vi "Error Codes List Window.vi"(5 "shift pressed?":bool, 7 "project file":path, 8 "error in (no error)":errorcluster, 9 "combo box text":string, 10 "scripting templates directory":path, 11 "project error file":path) -> ()   [LabVIEW 2017]
uses:
  Controls/Error Codes List Window Data.ctl
  Controls/Error Codes List Window States.ctl
  Controls/Quick Drop Input.ctl
  Controls/Error Codes List Window References.ctl
  Controls/Flags.ctl
  Error List/Scope.ctl
  Error List/Error Owner and ID.ctl
  <vilib>/Utility/miscctls.llb/LVRowAndColumnUnsignedTypeDef.ctl
  Controls/Themes.ctl
  Controls/Error Code Window Modes.ctl
  <vilib>/Utility/SystemLogging/NI_SystemLogging.lvlib
  Error File Management/Error File Management.lvlib
panel:
  in  "error codes":i32(listbox)
  out "loading":u8(ring)
  in  "edit error":bool
  in  "add error":bool
  in  "remove error":bool
  in  "edit file":bool
  in  "scope":bool
  in  "cancel":bool
  in  "ok":bool
  in  "filter":bool
  in  "filter string":string
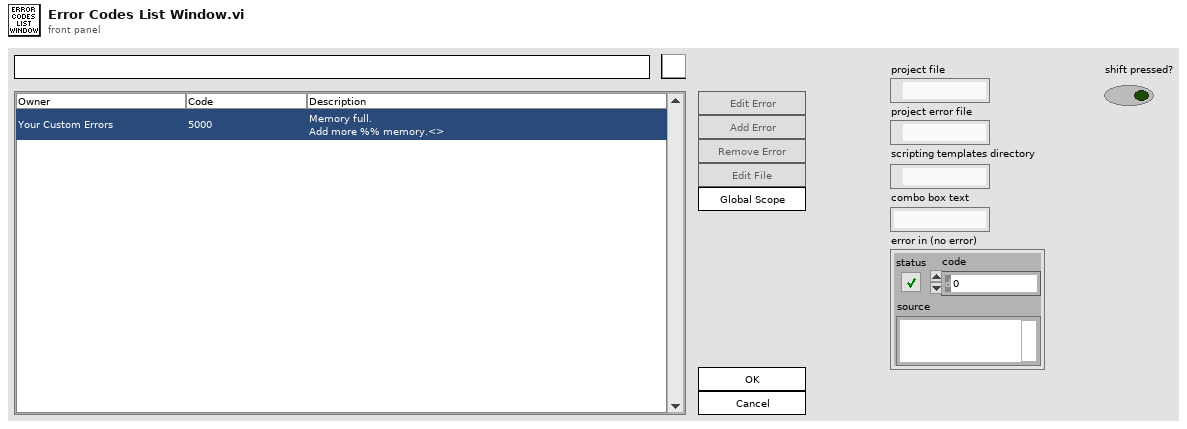
[diagram p1: front panel]
types:
  T1 = typedef "Error Codes List Window References.ctl" = cluster{"UI VI":refnum<vi>, "edit error":refnum<vi>, "add error":refnum<vi>, "remove error":refnum<vi>, "edit file":refnum<vi>, "scope":refnum<vi>, "ok":refnum<vi>, "cancel":refnum<vi>, "filter string":refnum<vi>, "filter":refnum<vi>, "error codes":refnum<vi>, "loading":refnum<vi>}
  T2 = typedef "Error Codes List Window Data.ctl" = cluster{"Q":refnum<queue>, "quick drop input":T3, "control references":T1, "flags":T4, "scope":T5, "error list":variant, "selected error":T6, "displayed errors":T6[]}
  T3 = typedef "Quick Drop Input.ctl" = cluster{"project file":path, "project error file":path, "scrip templates dir":path, "combo box string":string}
  T4 = typedef "Flags.ctl" = cluster{"place on cursor?":bool, "global scope loaded?":bool, "global modified?":bool, "filter on?":bool, "project scope avaiable?":bool, "shift pressed?":bool, "selected?":bool, "editable?":bool}
  T5 = typedef "Scope.ctl" = enum16{"project", "global"}
  T6 = typedef "Error Owner and ID.ctl" = cluster{"owner path":string, "ID":string}
  T7 = typedef "Error Codes List Window States.ctl" = enum16{"init", "load project errors", "parse combo box", "update list view", "open FP", "close", "idle", "add error", "remove error", "edit error", "edit file", "change scope", "filter"}
  T8 = enum32{"Invalid", "Standard", "Closed", "Hidden", "Minimized", "Maximized"}
  T9 = typedef "Themes.ctl" = enum16{"init", "edit buttons disable state", "loading on", "loading off", "scope name"}
  T10 = typedef "LVRowAndColumnUnsignedTypeDef.ctl" = cluster{"Row":u32, "Column":u32}
  T11 = typedef "Error File Management.lvlib/NI Error.ctl" = errorcluster
  T12 = typedef "LVPoint32TypeDef.ctl" = cluster{"Horizontal":i32, "Vertical":i32}
  T13 = typedef "Error Code Window Modes.ctl" = u8
  T14 = typedef "Error Code File Properties.ctl" = cluster{"path":path, "simplified path":string, "name":string, "display name":string, "family name":string, "comment":string, "parsable?":bool, "file modified?":bool}
  T15 = cluster{"new element/subarray":T14, "errors":T11[]}[]
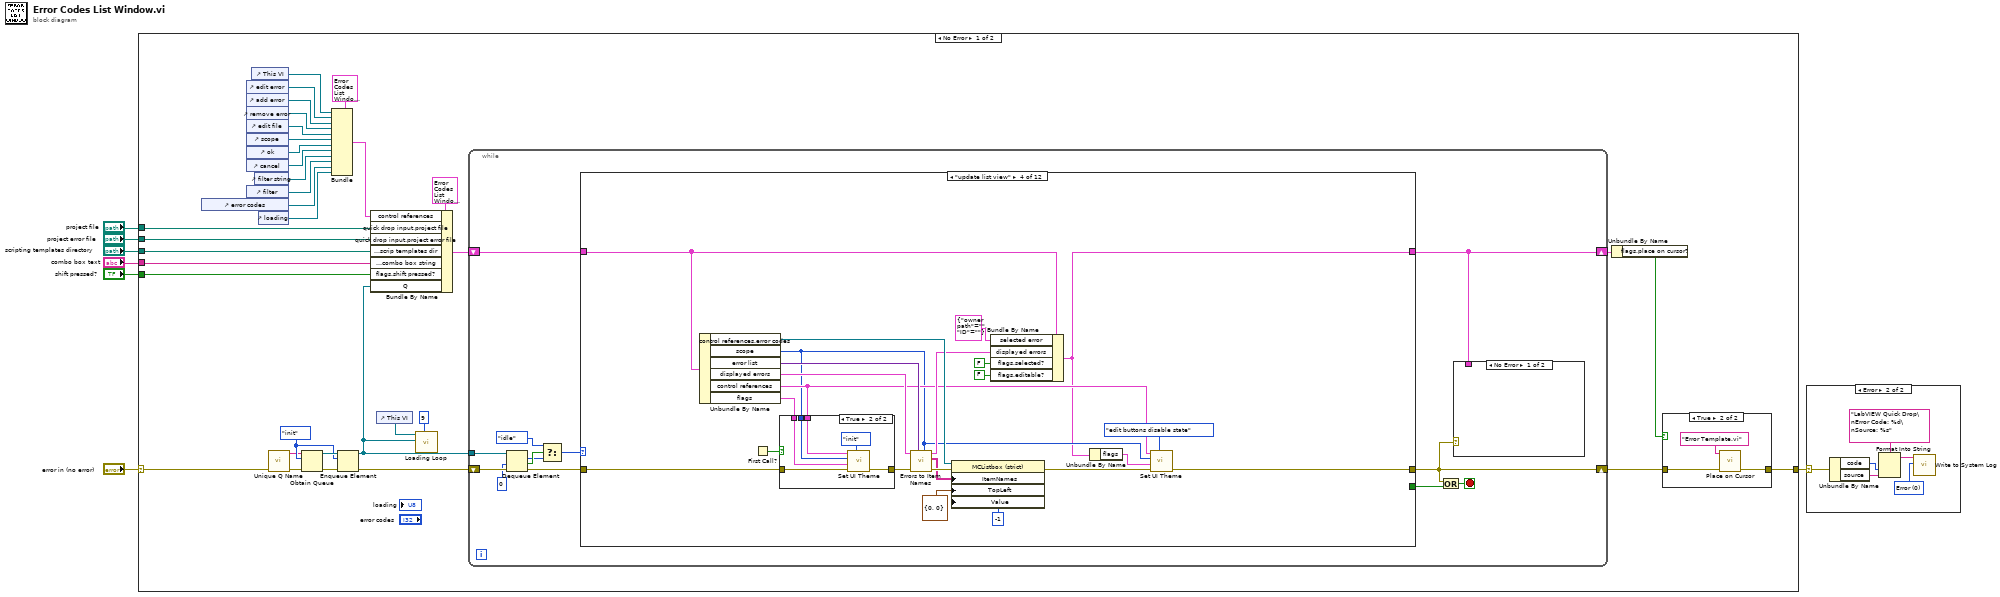
[diagram p0: block diagram]
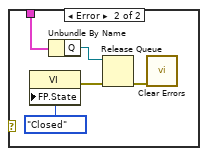
[diagram p2: hidden frame]
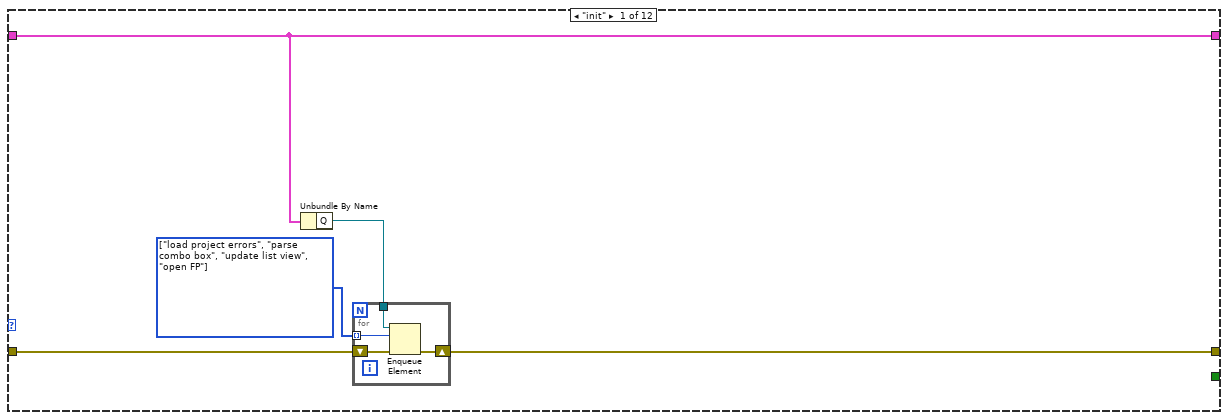
[diagram p3: hidden frame]
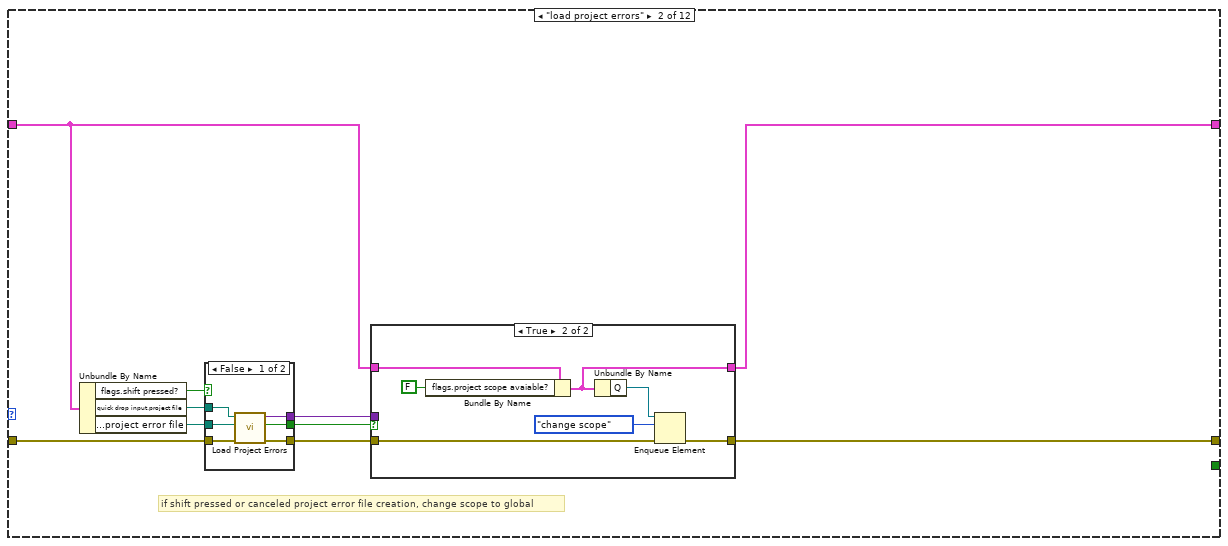
[diagram p4: hidden frame]
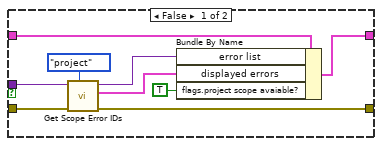
[diagram p6: hidden frame]
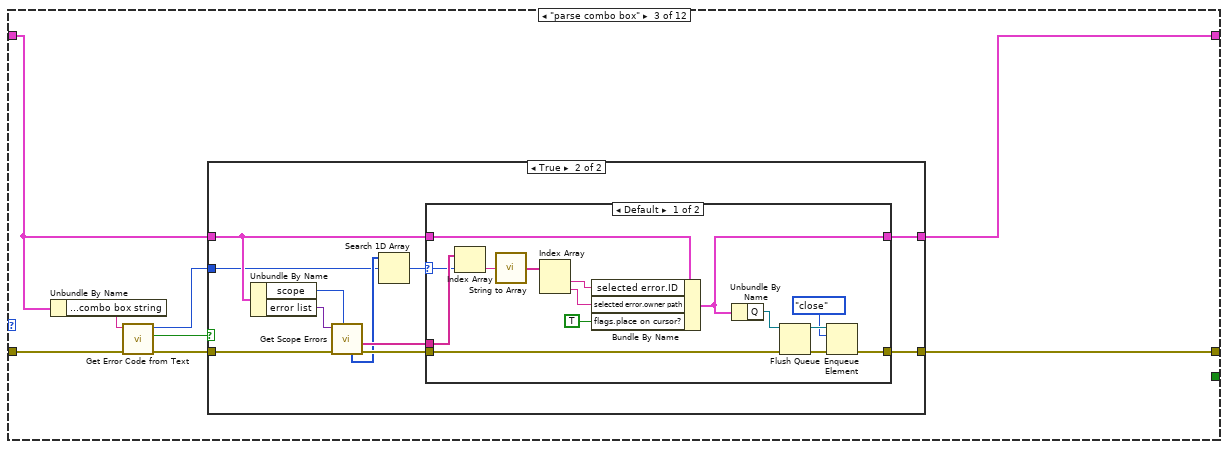
[diagram p7: hidden frame]
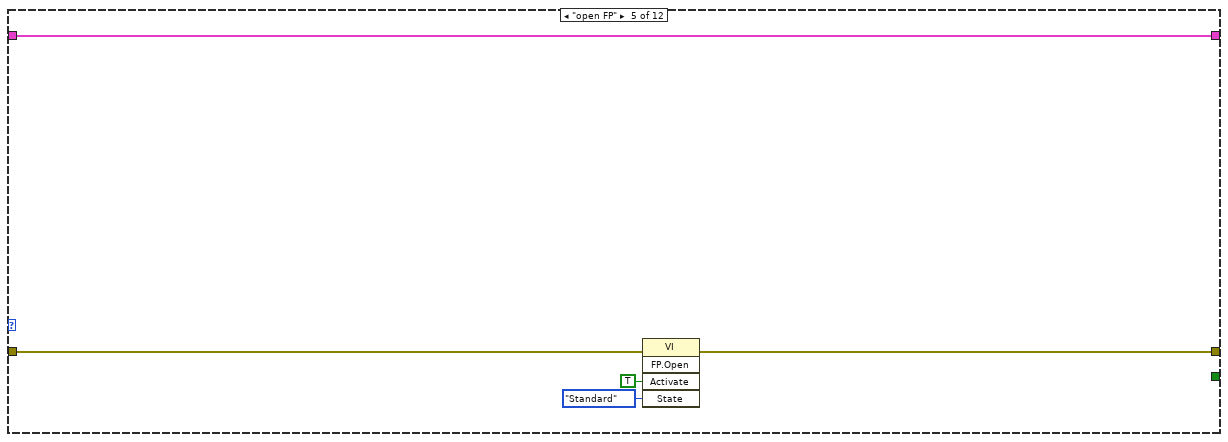
[diagram p11: hidden frame]
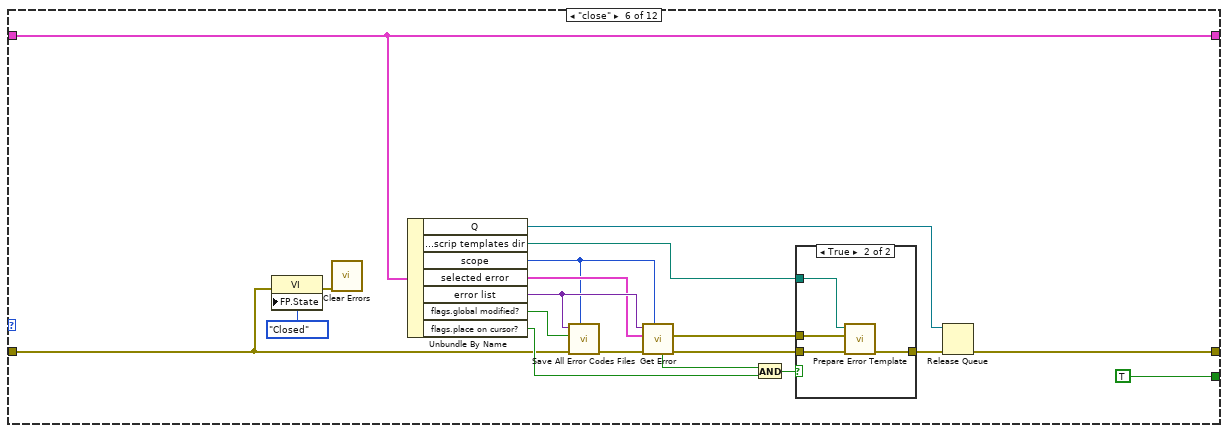
[diagram p12: hidden frame]
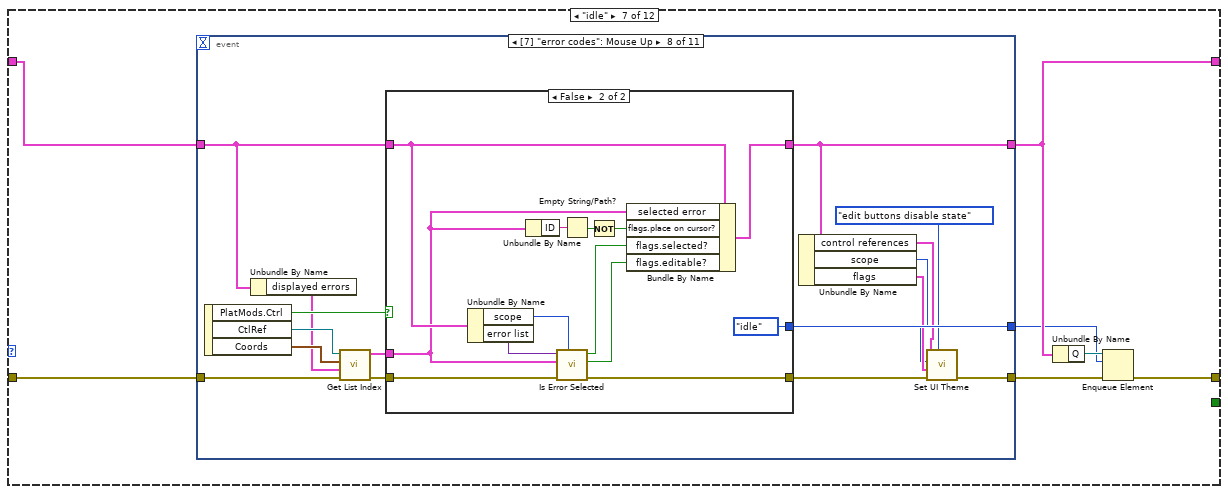
[diagram p14: hidden frame]
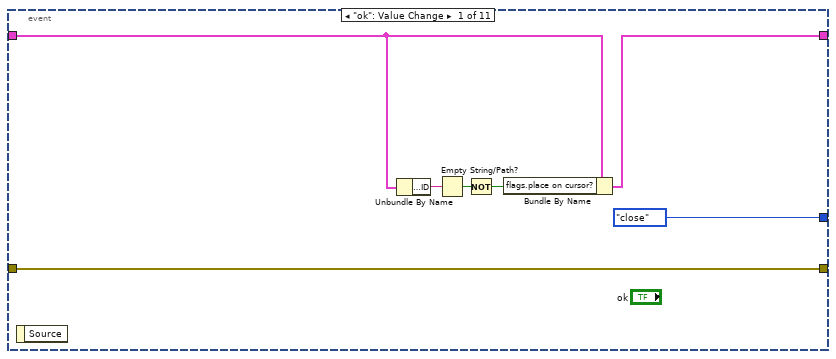
[diagram p15: hidden frame]
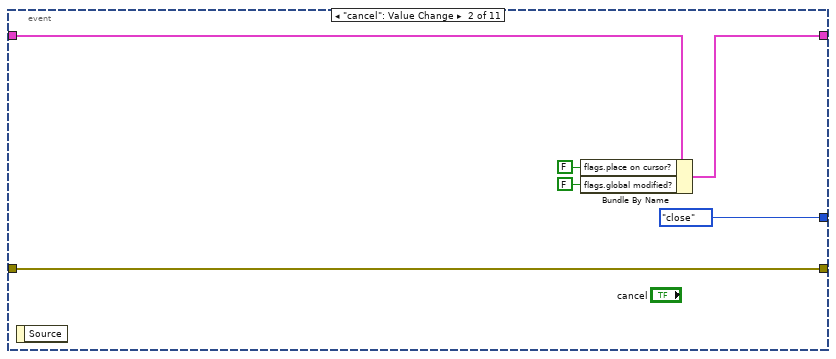
[diagram p16: hidden frame]
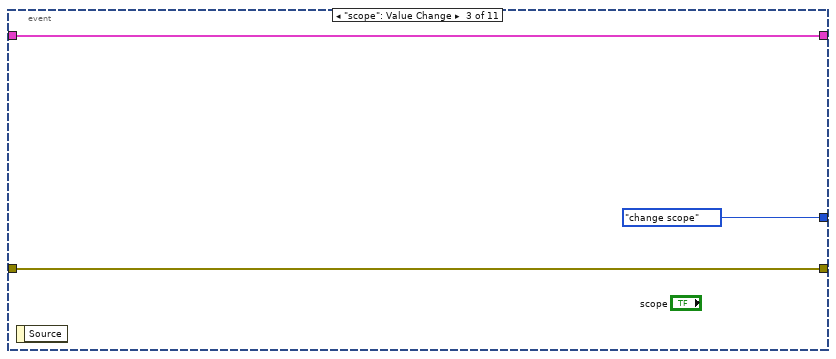
[diagram p17: hidden frame]
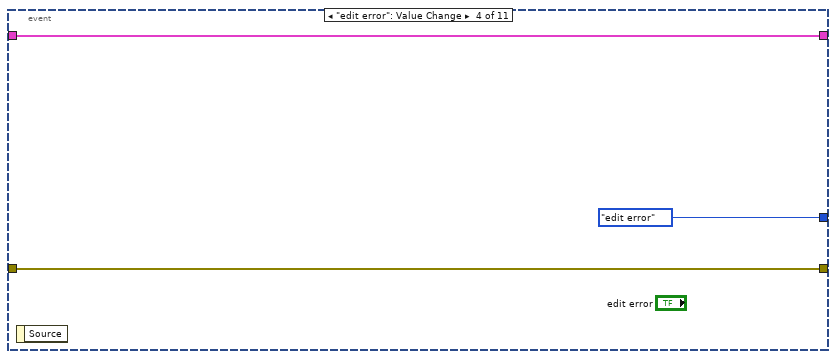
[diagram p18: hidden frame]
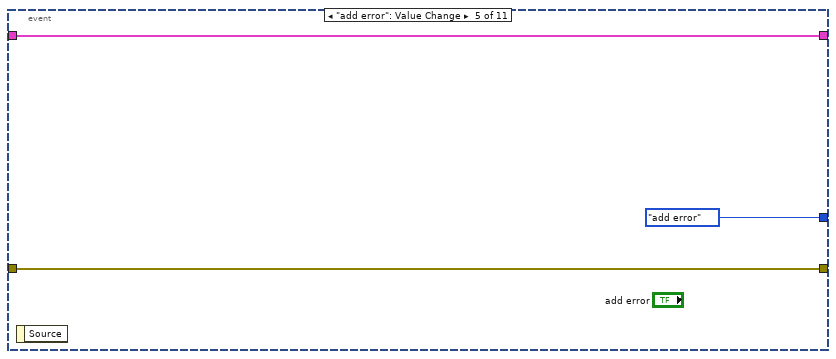
[diagram p19: hidden frame]
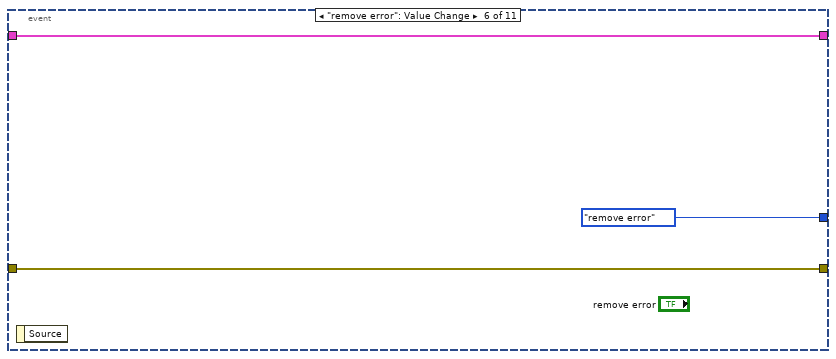
[diagram p20: hidden frame]
diagram:
  n1 = case shown="No Error" "error in (no error)" {
    selector: "error in (no error)" -> [w29 w440]
    tunnel: "project error file" -> [w12 _]
    tunnel: "scripting templates directory" -> [w27 _]
    tunnel: [w39 w440] -> w6
    tunnel: "combo box text" -> [w26 _]
    tunnel: "project file" -> [w11 _]
    tunnel: "shift pressed?" -> [w8 _]
    frame No Error {
      w30 = Error_Codes_List_Window_States."init" ("states")
      n2 = control-ref of="error codes"() -> (w15:refnum<vi>)
      n3 = control-ref of="edit error"() -> (w24:refnum<vi>)
      n4 = control-ref of="add error"() -> (w23:refnum<vi>)
      n5 = control-ref of="remove error"() -> (w22:refnum<vi>)
      n6 = control-ref of="edit file"() -> (w21:refnum<vi>)
      n7 = control-ref of="scope"() -> (w20:refnum<vi>)
      n8 = control-ref of="ok"() -> (w19:refnum<vi>)
      n9 = control-ref of="cancel"() -> (w18:refnum<vi>)
      n10 = control-ref of="filter"() -> (w16:refnum<vi>)
      n11 = control-ref of="This VI"() -> (w10:refnum<vi>)
      n12 = control-ref of="filter string"() -> (w17:refnum<vi>)
      n13 = control-ref of="loading"() -> (w14:refnum<vi>)
      n14 = call "Unique Q Name.vi"() -> ("unique Q name"=w28:string)  [unwired: 11 in]
      n15 = Obtain Queue(name (unnamed)=w28, element data type=w30, error in (no error)=w29) -> (queue out=w33:refnum<queue>, error out=w32:errorcluster)  [unwired: 2 in, 1 out]
      n16 = Bundle(cluster=T1 {"UI VI"=refnum, "edit error"=refnum, "add error"=refnum, "remove error"=refnum, "edit file"=refnum, "scope"=refnum, "ok"=refnum, "cancel"=refnum, "filter string"=refnum, "filter"=refnum, "error codes"=refnum, "loading"=refnum} ("control references"), "UI VI"=w10, "edit error"=w24, "add error"=w23, "remove error"=w22, "edit file"=w21, "scope"=w20, "ok"=w19, "cancel"=w18, "filter string"=w17, "filter"=w16, "error codes"=w15, "loading"=w14) -> (w13:T1)
      n17 = Enqueue Element(queue=w33, element=w30, error in (no error)=w32) -> (queue out=w25:refnum<queue>, error out=w31:errorcluster)  [unwired: 1 in, 1 out]
      n18 = Bundle By Name(cluster=T2 {"Q"=refnum, "quick drop input"={"project file"=path "", "project error file"=path "", "scrip templates dir"=path "", "combo box string"=""}, "control references"={"UI VI"=refnum, "edit error"=refnum, "add error"=refnum, "remove error"=refnum, "edit file"=refnum, "scope"=refnum, "ok"=refnum, "cancel"=refnum, "filter string"=refnum, "filter"=refnum, "error codes"=refnum, "loading"=refnum}, "flags"={"place on cursor?"=FALSE, "global scope loaded?"=FALSE, "global modified?"=FALSE, "filter on?"=FALSE, "project scope avaiable?"=FALSE, "shift pressed?"=FALSE, "selected?"=FALSE, "editable?"=FALSE}, "scope"=enum."project", "error list"=variant(cluster{"properties":cluster{"path":path, "simplified path":string, "name":string, "parsable?":bool, "project?":bool}, "data":cluster{"family":cluster{"family name":string, "display name":string}, "comment":string, "project errors":cluster{"error cluster":errorcluster, "owner file path":path, "owner display name":string, "parsable?":bool}[]}, "file modified?":bool}[] []), "selected error"={"owner path"="", "ID"=""}, "displayed errors"=[]} ("output cluster"), "control references"=w13, "quick drop input.project file"=w11, "quick drop input.project error file"=w12, "quick drop input.scrip templates dir"=w27, "quick drop input.combo box string"=w26, "flags.shift pressed?"=w8, "Q"=w25) -> (w40:T2)
      n19 = control-ref of="This VI"() -> (w35:refnum<vi>)
      n20 = call "Loading Loop.vi"("ctrl index"=9, "Q"=w25, "owner VI"=w35) -> ()  [unwired: 9 in]
      n21 = while {
        shift-right: [w43] -> w38
        shift-left: w31 -> [w51]
        shift-right: [w42] -> w37
        shift-left: w40 -> [w52]
        tunnel: w25 -> [w49]
        stop <- w53 stop-if-true
        n22 = Dequeue Element(queue=w49, timeout in ms (-1)=0, error in (no error)=w51) -> (element=w46:T7, timed out?=w47:bool, error out=w50:errorcluster)  [unwired: 1 out]
        n23 = Select(t=Error_Codes_List_Window_States."idle", s=w47, f=w46) -> (s? t:f=w45:T7)
        n24 = case shown="\"update list view\"" w45 {
          selector: w45 -> [_ _ _ _ _ _ _ _ w317 _ _ _]
          tunnel: [_ _ _ _ _ TRUE _ _ _ _ _ _] -> w54
          tunnel: w50 -> [w64 w78 w110 w158 w172 w179 w206 w311 w328 w351 w385 w421]
          tunnel: [w60 w70 w103 w148 w175 w192 w202 w301 w320 w339 w364 w411] -> w43
          tunnel: w52 -> [w63 w74 w106 w155 w171 w189 w205 w309 w327 w350 w384 w420]
          tunnel: [w63 w77 w105 w142 w171 w189 w201 w310 w326 w344 w378 w422] -> w42
          frame "init" {
            w61 = T7[] [enum."load project errors", enum."parse combo box", enum."update list view", enum."open FP"] items=["init", "load project errors", "parse combo box", "update list view", "open FP", "close", "idle", "add error", "remove error", "edit error", "edit file", "change scope", "filter"] ("t")
            n25 = Unbundle By Name(w63) -> ("Q"=w62:refnum<queue>)
            n26 = for {
              tunnel: w62 -> [w67]
              shift-right: [w68] -> w60
              shift-left: w64 -> [w66]
              tunnel: w61 -> [w65] mode=indexing
              n27 = Enqueue Element(queue=w67, element=w65, error in (no error)=w66) -> (error out=w68:errorcluster)  [unwired: 1 in, 2 out]
            }
          }
          frame "load project errors" {
            # "if shift pressed or canceled project error file creation, change scope to global"
            n28 = Unbundle By Name(w74) -> ("flags.shift pressed?"=w69:bool, "quick drop input.project file"=w72:path, "quick drop input.project error file"=w73:path)
            n29 = case shown="False" w69 {
              selector: w69 -> [_ w86]
              tunnel: w78 -> [w84 w85]
              tunnel: [w83 _] -> w76
              tunnel: [w82 w86] -> w75
              tunnel: w73 -> [w81 _]
              tunnel: w72 -> [w80 _]
              tunnel: [w79 w85] -> w71
              frame False {
                n30 = call "Load Project Errors.vi"("error in (no error)"=w84, "error file path"=w81, "project path"=w80) -> ("error out"=w79:errorcluster, "canceled?"=w82:bool, "error list <top>"=w83:variant)  [unwired: 6 in]
              }
              frame True {
              }
            }
            n31 = case shown="True" w75 {
              tunnel: [w95 w97] -> w77
              tunnel: w74 -> [w94 w98]
              tunnel: w76 -> [w93 _]
              tunnel: w71 -> [w91 w101]
              tunnel: [w90 w100] -> w70
              frame False {
                n32 = call "Get Scope Error IDs.vi"("scope"=Scope."project", "error in (no error)"=w91, "error list <top>"=w93) -> ("error out"=w90:errorcluster, "error IDs"=w89:T6[], "error list <top> dup"=w92:variant)  [unwired: 6 in]
                n33 = Bundle By Name(cluster=w94, "error list"=w92, "displayed errors"=w89, "flags.project scope avaiable?"=TRUE) -> (w95:T2)
              }
              frame True {
                n34 = Bundle By Name(cluster=w98, "flags.project scope avaiable?"=FALSE) -> (w97:T2)
                n35 = Unbundle By Name(w97) -> ("Q"=w102:refnum<queue>)
                n36 = Enqueue Element(queue=w102, element=Error_Codes_List_Window_States."change scope", error in (no error)=w101) -> (error out=w100:errorcluster)  [unwired: 1 in, 2 out]
              }
            }
          }
          frame "parse combo box" {
            n37 = Unbundle By Name(w106) -> ("quick drop input.combo box string"=w109:string)
            n38 = call "Get Error Code from Text.vi"("error in (no error)"=w110, "text"=w109) -> ("error out"=w104:errorcluster, "found?"=w108:bool, "code"=w107:i32)  [unwired: 7 in]
            n39 = case shown="True" w108 {
              tunnel: w107 -> [_ w113]
              tunnel: [w112 w122] -> w105
              tunnel: w106 -> [w112 w121]
              tunnel: w104 -> [w111 w118]
              tunnel: [w111 w119] -> w103
              frame False {
              }
              frame True {
                n40 = Unbundle By Name(w121) -> ("scope"=w115:T5, "error list"=w116:variant)
                n41 = call "Get Scope Errors.vi"("scope"=w115, "error in (no error)"=w118, "error list <top> in"=w116) -> ("error out"=w117:errorcluster, "attributes"=w123:string[], "error codes"=w114:i32[])  [unwired: 4 in, 2 out]
                n42 = Search 1D Array(1D array=w114, element=w113) -> (index of element=w120:i32)  [unwired: 1 in]
                n43 = case shown="Default" w120 {
                  selector: w120 -> [w128 _]
                  tunnel: [w133 w140] -> w122
                  tunnel: w121 -> [w137 w140]
                  tunnel: w117 -> [w132 w139]
                  tunnel: [w130 w139] -> w119
                  tunnel: w123 -> [w129 _]
                  frame Default {
                    n44 = Index Array(array=w129, index=w128) -> (element=w124:string)
                    n45 = call "String to Array.vi"("string"=w124) -> ("array"=w127:string[])  [unwired: 1 in]
                    n46 = Index Array(array=w127) -> (element #1=w126:string, element #2=w125:string)  [unwired: 2 in]
                    n47 = Bundle By Name(cluster=w137, "selected error.ID"=w126, "selected error.owner path"=w125, "flags.place on cursor?"=TRUE ("place on cursor?")) -> (w133:T2)
                    n48 = Unbundle By Name(w133) -> ("Q"=w136:refnum<queue>)
                    n49 = Flush Queue(queue=w136, error in (no error)=w132) -> (queue out=w135:refnum<queue>, error out=w131:errorcluster)  [unwired: 1 out]
                    n50 = Enqueue Element(queue=w135, element=Error_Codes_List_Window_States."close", error in (no error)=w131) -> (error out=w130:errorcluster)  [unwired: 1 in, 2 out]
                  }
                  frame -1 {
                  }
                }
              }
            }
          }
          frame "update list view" {
            n51 = Unbundle By Name(w155) -> ("control references.error codes"=w161:refnum<vi>, "scope"=w146:T5, "error list"=w159:variant, "displayed errors"=w160:T6[], "control references"=w147:T1, "flags"=w145:T4)
            n52 = First Call?() -> (First Call?: T/F=w151:bool)
            n53 = case shown="True" w151 {
              tunnel: w158 -> [w164 w170]
              tunnel: [w164 w169] -> w152
              tunnel: w146 -> [_ w168]
              tunnel: w147 -> [_ w167]
              tunnel: w145 -> [_ w166]
              frame False {
              }
              frame True {
                n54 = call "Set UI Theme.vi"("theme"=Themes."init", "error in (no error)"=w170, "flags"=w166, "global scope?"=w168, "control references"=w167) -> ("error out"=w169:errorcluster)  [unwired: 6 in]
              }
            }
            n55 = call "Errors to Item Names.vi"("scope"=w146, "error list <top>"=w159, "error in (no error)"=w152, "displayed errors in"=w160) -> ("error out"=w163:errorcluster, "item names"=w157:string[][], "displayed errors out"=w156:T6[])  [unwired: 5 in]
            n56 = property on="Property Node" class="MCListbox (strict)"(reference=w161, error in=w163, "ItemNames"=w157, "TopLeft"=T10 {"Row"=0, "Column"=0} ("Top Left Visible Cell"), "Value"=-1 ("error codes list")) -> (error out=w149:errorcluster)  [unwired: 1 out]
            n57 = Bundle By Name(cluster=w155, "selected error"=T6 {"owner path"="", "ID"=""}, "displayed errors"=w156, "flags.selected?"=FALSE, "flags.editable?"=FALSE) -> (w142:T2)
            n58 = Unbundle By Name(w142) -> ("flags"=w141:T4)
            n59 = call "Set UI Theme.vi"("theme"=Themes."edit buttons disable state", "error in (no error)"=w149, "flags"=w141, "global scope?"=w146, "control references"=w147) -> ("error out"=w148:errorcluster)  [unwired: 6 in]
          }
          frame "open FP" {
            n60 = invoke class="VI" method="FP.Open"(error in=w172, "Activate"=TRUE ("Activate?"), "State"=T8."Standard") -> (error out=w175:errorcluster)  [unwired: 2 in, 4 out]
          }
          frame "close" {
            n61 = property class="VI"(error in=w179, "FP.State"=T8."Closed" ("Front Panel Window:State")) -> (error out=w178:errorcluster)  [unwired: 1 in, 1 out]
            n62 = call <vilib>:"Clear Errors.vi"("error in (no error)"=w178) -> ()  [unwired: 5 in, 2 out]
            n63 = Unbundle By Name(w189) -> ("Q"=w191:refnum<queue>, "quick drop input.scrip templates dir"=w190:path, "scope"=w180:T5, "selected error"=w181:T6, "error list"=w184:variant, "flags.global modified?"=w187:bool, "flags.place on cursor?"=w183:bool)
            n64 = call "Save All Error Codes Files.vi"("scope"=w180, "error in (no error)"=w179, "save? (T)"=w187, "error list <top>"=w184) -> ("error out"=w186:errorcluster)  [unwired: 7 in]
            n65 = call "Get Error.vi"("scope"=w180, "error in (no error)"=w186, "owner error"=w181, "error list <top>"=w184) -> ("error out"=w185:errorcluster, "error"=w176:T11, "found?"=w177:bool)  [unwired: 3 in, 2 out]
            n66 = And(x=w177, y=w183) -> (x .and. y?=w182:bool)
            n67 = case shown="True" w182 {
              tunnel: w185 -> [w195 w199]
              tunnel: [w195 w198] -> w193
              tunnel: w190 -> [_ w197]
              tunnel: w176 -> [_ w196]
              frame False {
              }
              frame True {
                n68 = call "Prepare Error Template.vi"("error in (no error)"=w199, "error"=w196, "templates directory"=w197) -> ("error out"=w198:errorcluster)  [unwired: 8 in]
              }
            }
            n69 = Release Queue(queue=w191, error in (no error)=w193) -> (error out=w192:errorcluster)  [unwired: 1 in, 2 out]
          }
          frame "idle" {
            n70 = event shown="[7] \"error codes\": Mouse Up" {
              selector: _ -> [_ _ _ _ _ _ _ _ _ _ _]
              dyn-events: _ -> [_ _ _ _ _ _ _ _ _ _ _]
              timeout: _ -> [_ _ _ _ _ _ _ _ _ _ _]
              tunnel: w206 -> [w213 w217 w222 w225 w228 w231 w233 w249 w284 w290 w291]
              tunnel: [w213 w217 w222 w225 w228 w231 w233 w240 w284 w290 w291] -> w203
              tunnel: w205 -> [w210 w219 w221 w224 w227 w230 w234 w245 w280 w289 w295]
              tunnel: [w212 w218 w221 w224 w227 w230 w234 w238 w282 w289 w294] -> w201
              tunnel: [Error_Codes_List_Window_States."close" ("states") Error_Codes_List_Window_States."close" ("states") Error_Codes_List_Window_States."change scope" ("states") Error_Codes_List_Window_States."edit error" ("states") Error_Codes_List_Window_States."add error" ("states") Error_Codes_List_Window_States."remove error" ("states") Error_Codes_List_Window_States."edit file" ("states") w243 Error_Codes_List_Window_States."close" ("states") w285 Error_Codes_List_Window_States."filter" ("states")] -> w200
              event "ok": Value Change {
                n71 = event-data() -> ()  [unwired: 1 in, 1 out]
                n72 = Unbundle By Name(w210) -> ("selected error.ID"=w209:string)
                n73 = Empty String/Path?(string/path=w209) -> (empty?=w208:bool)
                n74 = Not(x=w208) -> (.not. x?=w207:bool)
                n75 = Bundle By Name(cluster=w210, "flags.place on cursor?"=w207) -> (w212:T2)
              }
              event "cancel": Value Change {
                n76 = event-data() -> ()  [unwired: 1 in, 1 out]
                n77 = Bundle By Name(cluster=w219, "flags.place on cursor?"=FALSE, "flags.global modified?"=FALSE) -> (w218:T2)
              }
              event "scope": Value Change {
                n78 = event-data() -> ()  [unwired: 1 in, 1 out]
              }
              event "edit error": Value Change {
                n79 = event-data() -> ()  [unwired: 1 in, 1 out]
              }
              event "add error": Value Change {
                n80 = event-data() -> ()  [unwired: 1 in, 1 out]
              }
              event "remove error": Value Change {
                n81 = event-data() -> ()  [unwired: 1 in, 1 out]
              }
              event "edit file": Value Change {
                n82 = event-data() -> ()  [unwired: 1 in, 1 out]
              }
              event "error codes": Mouse Up {
                n83 = event-data() -> ("PlatMods.Ctrl"=w250:bool, "CtlRef"=w247:refnum<vi>, "Coords"=w246:T12)  [unwired: 1 in]
                n84 = Unbundle By Name(w245) -> ("displayed errors"=w244:T6[])
                n85 = call "Get List Index.vi"("error in (no error)"=w249, "displayed errors"=w244, "coords"=w246, "error list"=w247) -> ("error out"=w242:errorcluster, "index"=w248:T6)  [unwired: 6 in]
                n86 = case shown="False" w250 {
                  tunnel: [w264 w266] -> w238
                  tunnel: w245 -> [w258 w275]
                  tunnel: w248 -> [w254 w267]
                  tunnel: [Error_Codes_List_Window_States."close" ("states") Error_Codes_List_Window_States."idle" ("states")] -> w243
                  tunnel: w242 -> [w260 w274]
                  tunnel: [w259 w276] -> w241
                  frame True {
                    n87 = Unbundle By Name(w254) -> ("ID"=w255:string)
                    n88 = Unbundle By Name(w258) -> ("scope"=w261:T5, "error list"=w262:variant)
                    n89 = Empty String/Path?(string/path=w255) -> (empty?=w251:bool)
                    n90 = call "Is Error Selected.vi"("global scope?"=w261, "error in (no error)"=w260, "selected error"=w254, "error codes files"=w262) -> ("error out"=w259:errorcluster, "editable?"=w256:bool, "selected?"=w257:bool)  [unwired: 5 in]
                    n91 = Compound Arithmetic op=AND(invert w251, TRUE ("value")) -> (w253:bool)
                    n92 = Bundle By Name(cluster=w258, "selected error"=w254, "flags.place on cursor?"=w253, "flags.selected?"=w257, "flags.editable?"=w256) -> (w264:T2)
                  }
                  frame False {
                    n93 = Unbundle By Name(w275) -> ("scope"=w265:T5, "error list"=w270:variant)
                    n94 = Unbundle By Name(w267) -> ("ID"=w273:string)
                    n95 = call "Is Error Selected.vi"("global scope?"=w265, "error in (no error)"=w274, "selected error"=w267, "error codes files"=w270) -> ("error out"=w276:errorcluster, "editable?"=w268:bool, "selected?"=w269:bool)  [unwired: 5 in]
                    n96 = Empty String/Path?(string/path=w273) -> (empty?=w272:bool)
                    n97 = Not(x=w272) -> (.not. x?=w271:bool)
                    n98 = Bundle By Name(cluster=w275, "selected error"=w267, "flags.place on cursor?"=w271, "flags.selected?"=w269, "flags.editable?"=w268) -> (w266:T2)
                  }
                }
                n99 = Unbundle By Name(w238) -> ("control references"=w235:T1, "scope"=w236:T5, "flags"=w237:T4)
                n100 = call "Set UI Theme.vi"("theme"=Themes."edit buttons disable state", "error in (no error)"=w241, "flags"=w237, "global scope?"=w236, "control references"=w235) -> ("error out"=w240:errorcluster)  [unwired: 6 in]
              }
              event Panel Close? {
                n101 = event-data() -> ()  [unwired: 1 in, 1 out]
                n102 = Bundle By Name(cluster=w280, "flags.place on cursor?"=FALSE ("place on cursor?"), "flags.global modified?"=FALSE ("modified?")) -> (w282:T2)
                n103 = event-data("Discard?"=TRUE) -> ()  [unwired: 1 in, 1 out]
              }
              event "filter string": Value Change {
                n104 = event-data() -> ()  [unwired: 1 in, 1 out]
                n105 = Unbundle By Name(w289) -> ("flags.filter on?"=w288:bool)
                n106 = Select(t=Error_Codes_List_Window_States."filter" ("states"), s=w288, f=Error_Codes_List_Window_States."idle" ("states")) -> (s? t:f=w285:T7)
              }
              event "filter": Value Change {
                n107 = event-data() -> ("NewVal"=w292:bool)  [unwired: 1 in]
                n108 = case shown="False" w292 {
                  frame False {
                    n109 = local write "filter string"("") -> ()
                  }
                  frame True {
                  }
                }
                n110 = Bundle By Name(cluster=w295, "flags.filter on?"=w292) -> (w294:T2)
              }
            }
            n111 = Unbundle By Name(w201) -> ("Q"=w204:refnum<queue>)
            n112 = Enqueue Element(queue=w204, element=w200, error in (no error)=w203) -> (error out=w202:errorcluster)  [unwired: 1 in, 2 out]
          }
          frame "remove error" {
            n113 = Unbundle By Name(w309) -> ("scope"=w298:T5, "error list"=w307:variant, "selected error"=w306:T6, "Q"=w304:refnum<queue>)
            n114 = Enqueue Element(queue=w304, element=Error_Codes_List_Window_States."update list view", error in (no error)=w311) -> (error out=w305:errorcluster)  [unwired: 1 in, 2 out]
            n115 = call "Remove Error.vi"("scope"=w298, "error in (no error)"=w305, "selected error"=w306, "error list <top> in"=w307) -> ("error out"=w302:errorcluster, "error list <top> out"=w300:variant)  [unwired: 6 in]
            n116 = call "Get Scope Error IDs.vi"("scope"=w298, "error in (no error)"=w302, "error list <top>"=w300) -> ("error out"=w301:errorcluster, "error IDs"=w297:T6[], "error list <top> dup"=w299:variant)  [unwired: 6 in]
            n117 = Bundle By Name(cluster=w309, "flags.global modified?"=TRUE, "error list"=w299, "displayed errors"=w297) -> (w310:T2)
          }
          frame "add error", "edit error" {
            w313 = T13 1 items=["create", "edit"] ("mode")
            w314 = T13 0 items=["create", "edit"] ("mode")
            n118 = Unbundle By Name(w327) -> ("Q"=w322:refnum<queue>, "error list"=w325:variant, "scope"=w324:T5, "selected error"=w323:T6)
            n119 = Equal?(x=w317, y=Error_Codes_List_Window_States."add error") -> (x = y?=w315:bool)
            n120 = Select(t=w314, s=w315, f=w313) -> (s? t:f=w312:T13)
            n121 = call "Error Code Window.vi"("mode"=w312, "error in (no error)"=w328, "selected error index"=w323, "scope"=w324, "error list <top> in"=w325) -> ("error out"=w321:errorcluster, "modified?"=w319:bool, "error list <top> out"=w318:variant)  [unwired: 4 in]
            n122 = case shown="True" w319 {
              tunnel: w327 -> [w330 w338]
              tunnel: [w330 w337] -> w326
              tunnel: w322 -> [_ w335]
              tunnel: w321 -> [w329 w334]
              tunnel: [w329 w333] -> w320
              tunnel: w318 -> [_ w332]
              frame False {
              }
              frame True {
                n123 = Bundle By Name(cluster=w338, "error list"=w332, "flags.global modified?"=TRUE) -> (w337:T2)
                n124 = Enqueue Element(queue=w335, element=Error_Codes_List_Window_States."update list view", error in (no error)=w334) -> (error out=w333:errorcluster)  [unwired: 1 in, 2 out]
              }
            }
          }
          frame "edit file" {
            w346 = T13 1 items=["create", "edit"] ("mode")
            n125 = Unbundle By Name(w350) -> ("Q"=w341:refnum<queue>, "scope"=w348:T5, "error list"=w349:variant, "selected error.owner path"=w347:string)
            n126 = call "Error Codes File Window.vi"("mode"=w346, "scope"=w348, "error in (no error)"=w351, "owner path"=w347, "error list <top> in"=w349) -> ("error out"=w340:errorcluster, "cancelled?"=w345:bool, "modified?"=w343:bool, "error list <top> out"=w342:variant)  [unwired: 3 in]
            n127 = case shown="False" w345 {
              tunnel: [w359 w361] -> w344
              tunnel: w350 -> [w358 w361]
              tunnel: w343 -> [w357 _]
              tunnel: w342 -> [w356 _]
              tunnel: w341 -> [w355 _]
              tunnel: w340 -> [w354 w360]
              tunnel: [w353 w360] -> w339
              frame False {
                n128 = Bundle By Name(cluster=w358, "error list"=w356, "flags.global modified?"=w357) -> (w359:T2)
                n129 = Enqueue Element(queue=w355, element=Error_Codes_List_Window_States."update list view", error in (no error)=w354) -> (error out=w353:errorcluster)  [unwired: 1 in, 2 out]
              }
              frame True {
              }
            }
          }
          frame "change scope" {
            n130 = Unbundle By Name(w384) -> ("control references"=w366:T1, "flags"=w365:T4)
            n131 = call "Set UI Theme.vi"("theme"=Themes."loading on", "error in (no error)"=w385, "flags"=w365, "control references"=w366) -> ("error out"=w386:errorcluster)  [unwired: 7 in]
            n132 = Unbundle By Name(w384) -> ("scope"=w363:T5, "flags.global scope loaded?"=w380:bool, "error list"=w382:variant, "displayed errors"=w371:T6[], "Q"=w376:refnum<queue>)
            n133 = Enqueue Element(queue=w376, element=Error_Codes_List_Window_States."update list view", error in (no error)=w386) -> (error out=w377:errorcluster)  [unwired: 1 in, 2 out]
            n134 = Not Equal To 0?(x=w363) -> (x != 0?=w373:bool)
            n135 = Not(x=w373) -> (.not. x?=w372:bool)
            n136 = Boolean To (0,1)(Boolean=w372) -> (0, 1=w362:i16)
            n137 = case shown="True" w380 {
              selector: w380 -> [w396 w405]
              tunnel: w377 -> [w398 w404]
              tunnel: [w391 w403] -> w383
              tunnel: w382 -> [w393 w402]
              tunnel: [w388 w401] -> w381
              tunnel: [w397 w405] -> w379
              tunnel: w371 -> [_ _]
              tunnel: [w387 w400] -> w370
              tunnel: w362 -> [_ w399]
              frame False {
                w389 = Scope."global" ("scope")
                # "load errors"
                n138 = call "Load Built-in Error Codes.vi"("error in (no error)"=w398) -> ("error out"=w394:errorcluster, "error codes files content"=w395:T15)  [unwired: 9 in]
                n139 = call "Insert Scope Errors.vi"("scope"=w389, "error in (no error)"=w394, "error codes file content"=w395, "error list <top> in"=w393) -> ("error out"=w392:errorcluster, "error list <top> out"=w390:variant)  [unwired: 6 in]
                n140 = Not(x=w396) -> (.not. x?=w397:bool)
                n141 = call "Get Scope Error IDs.vi"("scope"=w389, "error in (no error)"=w392, "error list <top>"=w390) -> ("error out"=w391:errorcluster, "error IDs"=w387:T6[], "error list <top> dup"=w388:variant)  [unwired: 6 in]
              }
              frame True {
                # "already loaded"
                n142 = call "Get Scope Error IDs.vi"("scope"=w399, "error in (no error)"=w404, "error list <top>"=w402) -> ("error out"=w403:errorcluster, "error IDs"=w400:T6[], "error list <top> dup"=w401:variant)  [unwired: 6 in]
              }
            }
            n143 = Bundle By Name(cluster=w384, "scope"=w362, "flags.global scope loaded?"=w379, "error list"=w381, "displayed errors"=w370) -> (w378:T2)
            n144 = call "Set UI Theme.vi"("theme"=Themes."loading off", "error in (no error)"=w383, "flags"=w365, "control references"=w366) -> ("error out"=w368:errorcluster)  [unwired: 7 in]
            n145 = call "Set UI Theme.vi"("theme"=Themes."scope name", "error in (no error)"=w368, "global scope?"=w362, "control references"=w366) -> ("error out"=w364:errorcluster)  [unwired: 7 in]
          }
          frame "filter" {
            # "#TODO add display name based filtering, only parsable filtering,\nduplicates, file name filtering"
            n146 = Unbundle By Name(w420) -> ("scope"=w407:T5, "error list"=w414:variant, "displayed errors"=w415:T6[], "Q"=w417:refnum<queue>, "control references"=w409:T1, "flags"=w408:T4)
            n147 = call "Set UI Theme.vi"("theme"=Themes."loading on", "error in (no error)"=w421, "flags"=w408, "global scope?"=w407, "control references"=w409) -> ("error out"=w412:errorcluster)  [unwired: 6 in]
            n148 = Enqueue Element(queue=w417, element=Error_Codes_List_Window_States."update list view", error in (no error)=w412) -> (error out=w423:errorcluster)  [unwired: 1 in, 2 out]
            n149 = case shown="Default" "filter string" {
              selector: "filter string" -> [_ w429]
              tunnel: w423 -> [w428 w435]
              tunnel: [w424 w434] -> w419
              tunnel: [w425 w433] -> w418
              tunnel: w415 -> [_ w432]
              tunnel: w414 -> [w427 w431]
              tunnel: w407 -> [w426 w430]
              frame "" {
                n150 = call "Get Scope Error IDs.vi"("scope"=w426, "error in (no error)"=w428, "error list <top>"=w427) -> ("error out"=w424:errorcluster, "error IDs"=w425:T6[])  [unwired: 6 in, 1 out]
              }
              frame Default {
                n151 = call "Filter.vi"("scope"=w430, "error list"=w431, "error in (no error)"=w435, "filter string"=w429, "displayed errors in"=w432) -> ("error out"=w434:errorcluster, "displayed errors out"=w433:T6[])  [unwired: 5 in]
              }
            }
            n152 = Bundle By Name(cluster=w420, "displayed errors"=w418) -> (w422:T2)
            n153 = call "Set UI Theme.vi"("theme"=Themes."loading off", "error in (no error)"=w419, "flags"=w408, "global scope?"=w407, "control references"=w409) -> ("error out"=w411:errorcluster)  [unwired: 6 in]
          }
        }
        n154 = Or(x=w43, y=w54) -> (x .or. y?=w53:bool)
        n155 = case shown="No Error" w43 {
          tunnel: w42 -> [_ w59]
          frame No Error {
          }
          frame Error {
            n156 = property class="VI"("FP.State"=T8."Closed" ("Front Panel Window:State")) -> (error out=w56:errorcluster)  [unwired: 2 in, 1 out]
            n157 = Unbundle By Name(w59) -> ("Q"=w58:refnum<queue>)
            n158 = Release Queue(queue=w58, error in (no error)=w56) -> (error out=w55:errorcluster)  [unwired: 1 in, 2 out]
            n159 = call <vilib>:"Clear Errors.vi"("error in (no error)"=w55) -> ()  [unwired: 5 in, 2 out]
          }
        }
      }
      n160 = Unbundle By Name(w37) -> ("flags.place on cursor?"=w36:bool)
      n161 = case shown="True" w36 {
        tunnel: [w436 w439] -> w39
        tunnel: w38 -> [w436 w438]
        frame False {
        }
        frame True {
          n162 = call "Place on Cursor.vi"("error in (no error)"=w438, "name"="Error Template.vi") -> ("error out"=w439:errorcluster)  [unwired: 8 in, 1 out]
        }
      }
    }
    frame Error {
    }
  }
  n163 = case shown="Error" w6 {
    selector: w6 -> [_ w445]
    frame No Error {
    }
    frame Error {
      w446 = 0 items=["Error", "Warning", "Informational"] ("severity")
      n164 = Unbundle By Name(w445) -> ("code"=w442:i32, "source"=w441:string)
      n165 = Format Into String(format string="LabVIEW Quick Drop\nError Code: %d\nSource: %s", w442, w441) -> (resulting string=w443:string)  [unwired: 2 in, 1 out]
      n166 = call <vilib>:"Write to System Log.vi"("severity"=w446, "message"=w443) -> ()  [unwired: 9 in, 1 out]
    }
  }
